vi "Voltage Update.vi"(0 "Voltage Output":dbl(slide) scale=-10.0..9.995 scale format="%.3f", 2 "Physical Channel":tag="PXI1Slot7/ao0") -> ()   [LabVIEW 2016, in "Transport.lvclass"]
doc: "I. Description:\nThis example demonstrates how to output a single Voltage Update (Sample) to an Analog Output Channel.\n\nII. Instructions for Running:\n1. Select the Physical Channel to correspond to where your signal is output on the DAQ device.\n2. Enter the Minimum and Maximum Voltage Ranges\nNote: Use the Acq One Sample example to verify you are generating the correct output on the DAQ device\n\nIII. Block Diagram Steps:\n1. Create an Analog Output Voltage Channel\n2. Use the Write VI to Output 1 Sample to 1 Channel on the Data\nAcquisition Card. \n3. Call the Clear Task VI to clear the Task.\n4. Use the popup dialog box to display an error if any. \n\nIV. I/O Connections Overview:\nMake sure your signal output terminal matches the Physical Channel I/O Control. For further connection information, refer to your hardware reference manual."
uses:
  Transport.lvclass
  <vilib>/Utility/error.llb/DialogType.ctl
  <vilib>/DAQmx/write.llb/DAQmx Write (Analog DBL 1Chan 1Samp).vi
  <vilib>/DAQmx/create/channels.llb/DAQmx Create Channel (AO-Voltage-Basic).vi
  <vilib>/DAQmx/configure/timing.llb/DAQmx Timing (Sample Clock).vi
  <vilib>/DAQmx/miscellaneous.llb/DAQmx Fill In Error Info.vi
  <resource>/objmgr/daqmx.rc
panel:
  in  "gain":dbl
  in  "Maximum Value":dbl=10.0 format="%0.2f"
  in  "Minimum Value":dbl=-10.0 format="%0.2f"
  # "For instructions, select Help>>Show Context Help"
  # "Channel Parameters"
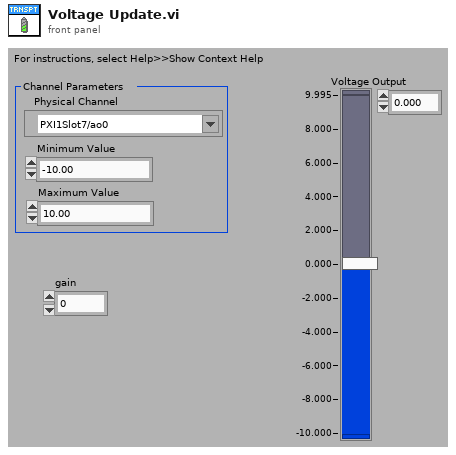
[diagram p1: front panel]
types:
  T1 = typedef "DialogType.ctl" = u16
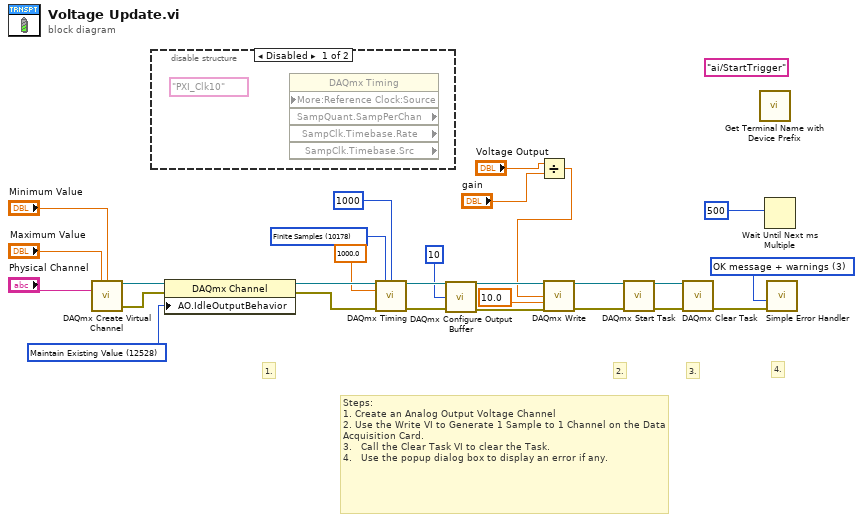
[diagram p0: block diagram]
diagram:
  (unwired) "ai/StartTrigger" ("Local Terminal Name")
  w5 = 10178 items=["Finite Samples"=10178, "Continuous Samples"=10123, "Hardware Timed Single Point"=12522] ("sample mode")
  w19 = 12528 items=["Zero Volts"=12526, "High-Impedance"=12527, "Maintain Existing Value"=12528] ("AO.IdleOutputBehavior")
  w24 = T1 3 items=["no dialog", "OK message", "continue or stop message", "OK message + warnings", "continue/stop + warnings"] ("type of dialog (OK msg:1)")
  # "4."
  # "2."
  # "Steps: \n1. Create an Analog Output Voltage Channel\n2. Use the Write VI to Generate 1 Sample to 1 Channel on the Data Acquisition Card.  \n3.   Call the Clear Task VI to clear the Task.\n4.   Use the popup dialog box to display an error if any."
  # "3."
  # "1."
  n1 = call-poly <vilib>:"DAQmx Create Virtual Channel.vi"("maximum value"="Maximum Value", "minimum value"="Minimum Value", "physical channels"="Physical Channel") -> ("task out"=w21:refnum<k21>, "error out"=w20:errorcluster)  [unwired: 11 in]
  n2 = disable-structure shown="Disabled" {
    frame Disabled {
      (unwired) tag "PXI_Clk10" ("RefClk.Src")
      n3 = property class="DAQmx Timing" props=["More:Reference Clock:Source", "SampQuant.SampPerChan", "SampClk.Timebase.Rate", "SampClk.Timebase.Src"]() -> ()  [unwired: 3 in, 5 out]
    }
    frame Enabled {
    }
  }
  n4 = property class="DAQmx Channel"(reference=w21, error in=w20, "AO.IdleOutputBehavior"=w19) -> (reference out=w17:refnum<k21>, error out=w16:errorcluster)
  n5 = call-poly <vilib>:"DAQmx Timing.vi"("task/channels in"=w17, "sample mode"=w5, "samples per channel"=1000, "rate"=1000.0, "error in"=w16) -> ("task out"=w10:refnum<k21>, "error out"=w9:errorcluster)  [unwired: 9 in]
  n6 = call <vilib>:"DAQmx Configure Output Buffer.vi"("task/channels in"=w10, "buffer size (in samples per channel)"=u32 10, "error in"=w9) -> ("task out"=w7:refnum<k21>, "error out"=w8:errorcluster)  [unwired: 11 in]
  n7 = Divide(x="Voltage Output", y="gain") -> (x/y=w2:dbl)
  n8 = call-poly <vilib>:"DAQmx Write.vi"("task/channels in"=w7, "data"=w2, "timeout"=10.0, "error in"=w8) -> ("task out"=w11:refnum<k21>, "error out"=w12:errorcluster)  [unwired: 9 in, 1 out]
  n9 = call <vilib>:"DAQmx Start Task.vi"("task/channels in"=w11, "error in"=w12) -> ("task out"=w14:refnum<k21>, "error out"=w13:errorcluster)  [unwired: 12 in]
  n10 = call <vilib>:"DAQmx Clear Task.vi"("task in"=w14, "error in"=w13) -> ("error out"=w23:errorcluster)  [unwired: 13 in]
  n11 = call <userlib>:"Get Terminal Name with Device Prefix.vi"() -> ()  [unwired: 9 in, 3 out]
  n12 = Wait Until Next ms Multiple(millisecond multiple=u32 500 ("milliseconds to wait")) -> ()  [unwired: 1 out]
  n13 = call <vilib>:"Simple Error Handler.vi"("type of dialog (OK msg:1)"=w24, "error in (no error)"=w23) -> ()  [unwired: 3 in, 5 out]
